vi "svx_Colormap Create Menu Items.vi"() -> (1 "item tags":string[](array[string])=["USER_SC_AUTOSCALE_X", "USER_SC_AUTOSCALE_Y", "USER_SC_AUTOSCALE_Z", "USER_SC_IGNORE_COLOR_ARRAY", "USER_SC_INTERPOLATE_COLOR", "USER_SC_SMOOTH_UPDATES", "USER_SC_SCALE_LEGEND", "USER_SC_GRAPH_PALETTE", "USER_SC_CURSOR_LEGEND", "USER_SC_ORDER", "USER_SC_FREQ", "USER_SC_ADD"], 3 "menu items":T1(array[cluster])=[{"menu tag"="", "item names"="AutoScale X", "item tags"="USER_SC_AUTOSCALE_X"}, {"menu tag"="", "item names"="AutoScale Y", "item tags"="USER_SC_AUTOSCALE_Y"}, {"menu tag"="", "item names"="AutoScale Z", "item tags"="USER_SC_AUTOSCALE_Z"}, {"menu tag"="", "item names"="Ignore Color Array", "item tags"="USER_SC_IGNORE_COLOR_ARRAY"}, {"menu tag"="", "item names"="Interpolate Color", "item tags"="USER_SC_INTERPOLATE_COLOR"}, {"menu tag"="", "item names"="Smooth Updates", "item tags"="USER_SC_SMOOTH_UPDATES"}, {"menu tag"="", "item names"="-", "item tags"="APP_SC_SEPARATOR"}, {"menu tag"="", "item names"="Cursor Lines", "item tags"="USER_INDICATION_LINES"}, {"menu tag"="APP_SC_VISIBLE_ITEMS", "item names"="Scale Legend", "item tags"="USER_SC_SCALE_LEGEND"}, {"menu tag"="APP_SC_VISIBLE_ITEMS", "item names"="Graph Palette", "item tags"="USER_SC_GRAPH_PALETTE"}, {"menu tag"="APP_SC_VISIBLE_ITEMS", "item names"="Cursor Legend", "item tags"="USER_SC_CURSOR_LEGEND"}, {"menu tag"="USER_INDICATION_LINES", "item names"="Show Current Order", "item tags"="USER_SC_ORDER"}, {"menu tag"="USER_INDICATION_LINES", "item names"="Show Current Frequency", "item tags"="USER_SC_FREQ"}, {"menu tag"="USER_INDICATION_LINES", "item names"="Anchor Current", "item tags"="USER_SC_ADD"}, {"menu tag"="USER_INDICATION_LINES", "item names"="-", "item tags"="APP_SC_SEPARATOR_1"}, {"menu tag"="USER_INDICATION_LINES", "item names"="Customize...", "item tags"="USER_SC_CREATE_INDICATION_LINES"}, {"menu tag"="", "item names"="-", "item tags"="USER_SC_CREATE_INDICATION_LINES"}])   [LabVIEW 2017, in "SVX Colormap.xctl"]
uses:
  <vilib>/addons/_XControls/Colormap/SVX Colormap.xctl
panel:
  out "Backup":T1(array[cluster])=[{"menu tag"="", "item names"="Visible Items", "item tags"="APP_SC_VISIBLE_ITEMS"}, {"menu tag"="APP_SC_VISIBLE_ITEMS", "item names"="Label", "item tags"="USER_SC_LABEL"}, {"menu tag"="APP_SC_VISIBLE_ITEMS", "item names"="Caption", "item tags"="USER_SC_CAPTION"}, {"menu tag"="APP_SC_VISIBLE_ITEMS", "item names"="-", "item tags"="APP_SEPARATOR"}, {"menu tag"="APP_SC_VISIBLE_ITEMS", "item names"="Scale Legend", "item tags"="APP_SC_SCALE_LEGEND"}, {"menu tag"="APP_SC_VISIBLE_ITEMS", "item names"="Graph Palette", "item tags"="APP_SC_GRAPH_PALETTE"}, {"menu tag"="APP_SC_VISIBLE_ITEMS", "item names"="Cursor Legend", "item tags"="APP_SC_CURSOR_LEGEND"}, {"menu tag"="APP_SC_VISIBLE_ITEMS", "item names"="X Scrollbar", "item tags"="APP_SC_X_SCROLLBAR"}, {"menu tag"="", "item names"="Reinitialize to Default Value", "item tags"="APP_SC_REINIT_TO_DEFAULT_VALUE"}, {"menu tag"="", "item names"="-", "item tags"="APP_SEPARATOR"}, {"menu tag"="", "item names"="Description and Tip...", "item tags"="APP_SC_DESCRIPTION_AND_TIP"}, {"menu tag"="", "item names"="-", "item tags"="APP_SEPARATOR"}, {"menu tag"="", "item names"="Clear Graph", "item tags"="APP_SC_CLEAR_GRAPH"}, {"menu tag"="", "item names"="Create Annotation", "item tags"="APP_SC_CREATE_ANNOTATION"}, {"menu tag"="", "item names"="Delete All Annotations", "item tags"="APP_SC_DELETE_ALL_ANNOTATIONS"}, {"menu tag"="", "item names"="-", "item tags"="APP_SEPARATOR"}, {"menu tag"="", "item names"="AutoScale X", "item tags"="APP_SC_AUTOSCALE_X"}, {"menu tag"="", "item names"="AutoScale Y", "item tags"="APP_SC_AUTOSCALE_Y"}, {"menu tag"="", "item names"="AutoScale Z", "item tags"="APP_SC_AUTOSCALE_Z"}, {"menu tag"="", "item names"="Ignore Color Array", "item tags"="APP_SC_IGNORE_COLOR_ARRAY"}, {"menu tag"="", "item names"="Interpolate Color", "item tags"="APP_SC_INTERPOLATE_COLOR"}, {"menu tag"="", "item names"="Smooth Updates", "item tags"="APP_SC_SMOOTH_UPDATES"}]
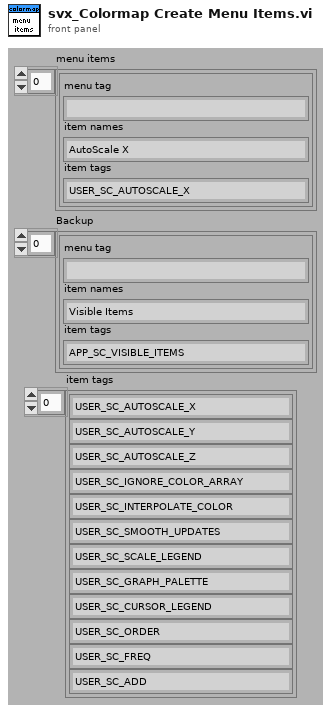
[diagram p1: front panel]
types:
  T1 = cluster{"menu tag":string, "item names":string, "item tags":string}[]
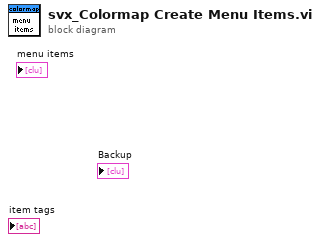
[diagram p0: block diagram]
diagram:
